vi "Curtin1_ReadWriteView.vi"(8 "X_High":dbl, 9 "X_Low":dbl, 11 "Task":enum16{"Read", "Save"}(ring)) -> (0 "X_High out":dbl, 1 "X_Low out":dbl, 3 "View":T1={"Alerts"=FALSE, "Log X Axis"=TRUE, "dB scale"=TRUE, "Averaging"=TRUE, "Fade"=0.8181818181818182, "Centroids?"=TRUE})   [LabVIEW 2022 SP3]
uses:
  Mic/Mic_Global.vi
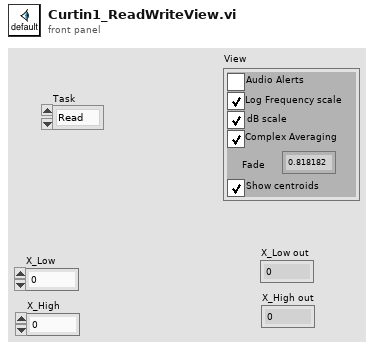
[diagram p1: front panel]
types:
  T1 = cluster{"Alerts":bool, "Log X Axis":bool, "dB scale":bool, "Averaging":bool, "Fade":dbl, "Centroids?":bool}
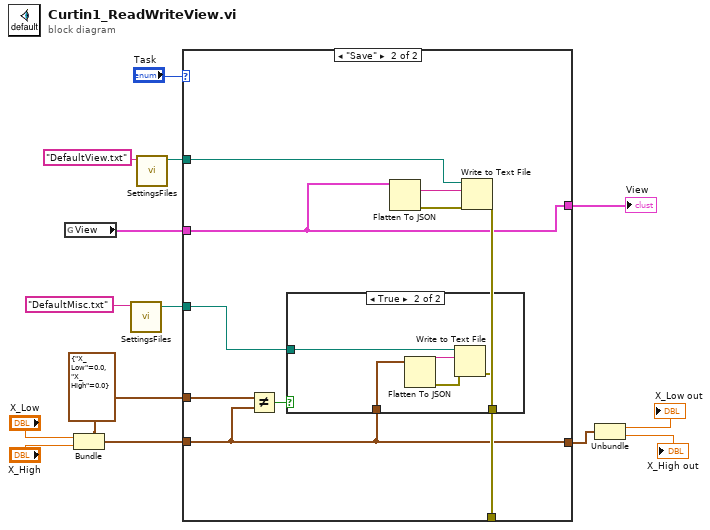
[diagram p0: block diagram]
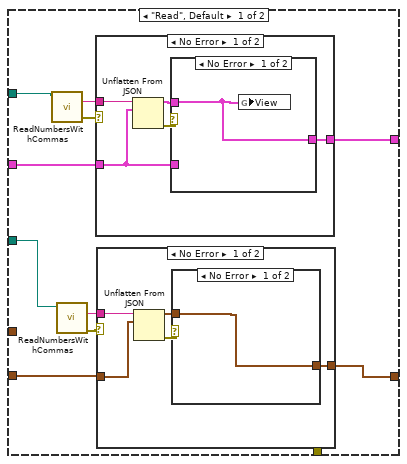
[diagram p2: hidden frame]
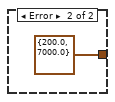
[diagram p3: hidden frame]
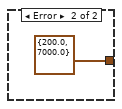
[diagram p4: hidden frame]
diagram:
  w6 = cluster{"X_Low":dbl, "X_High":dbl} {"X_Low"=0.0, "X_High"=0.0} ("output cluster")
  n1 = global read "Mic_Global.vi" "View"() -> (w10:T1)
  n2 = Bundle(cluster=w6, "X_Low"="X_Low", "X_High"="X_High") -> (w11:cluster{"X_Low":dbl, "X_High":dbl})
  n3 = call "SettingsFiles.vi"("settings file name"="DefaultMisc.txt" ("name or relative path")) -> ("file path"=w1:path)  [unwired: 9 in, 1 out]
  n4 = call "SettingsFiles.vi"("settings file name"="DefaultView.txt" ("name or relative path")) -> ("file path"=w3:path)  [unwired: 9 in, 1 out]
  n5 = case shown="\"Save\"" "Task" {
    tunnel: w3 -> [w17 w47]
    tunnel: [_ w46] -> _
    tunnel: w11 -> [w23 w42]
    tunnel: w10 -> [w24 w41]
    tunnel: w1 -> [w18 w45]
    tunnel: [w22 w42] -> w9
    tunnel: w6 -> [_ w43]
    tunnel: [w21 w41] -> w5
    frame "Read", Default {
      n6 = call "ReadNumbersWithCommas.vi"("file (use dialog)"=w17) -> ("error out"=w15:errorcluster, "text"=w16:string)  [unwired: 7 in, 2 out]
      n7 = call "ReadNumbersWithCommas.vi"("file (use dialog)"=w18) -> ("error out"=w20:errorcluster, "text"=w19:string)  [unwired: 7 in, 2 out]
      n8 = case shown="No Error" w15 {
        tunnel: w16 -> [w37 _]
        tunnel: w24 -> [w33 w40]
        tunnel: [w34 w40] -> w21
        frame No Error {
          n9 = Unflatten From JSON(JSON string=w37, type and defaults=w33) -> (value=w35:T1, error out=w36:errorcluster)  [unwired: 5 in]
          n10 = case shown="No Error" w36 {
            tunnel: w35 -> [w38 _]
            tunnel: [w38 w39] -> w34
            tunnel: w33 -> [_ w39]
            frame No Error {
              n11 = global write "Mic_Global.vi" "View"(w38) -> ()
            }
            frame Error {
            }
          }
        }
        frame Error {
        }
      }
      n12 = case shown="No Error" w20 {
        tunnel: w19 -> [w29 _]
        tunnel: w23 -> [w26 _]
        tunnel: [w25 cluster{"X_Low":dbl, "X_High":dbl} {"X_Low"=200.0, "X_High"=7000.0} ("output cluster")] -> w22
        frame No Error {
          n13 = Unflatten From JSON(JSON string=w29, type and defaults=w26) -> (value=w27:cluster{"X_Low":dbl, "X_High":dbl}, error out=w28:errorcluster)  [unwired: 5 in]
          n14 = case shown="No Error" w28 {
            tunnel: w27 -> [w30 _]
            tunnel: [w30 cluster{"X_Low":dbl, "X_High":dbl} {"X_Low"=200.0, "X_High"=7000.0} ("output cluster")] -> w25
            frame No Error {
            }
            frame Error {
            }
          }
        }
        frame Error {
        }
      }
    }
    frame "Save" {
      n15 = Not Equal?(x=w43, y=w42) -> (x != y?=w44:bool)
      n16 = case shown="True" w44 {
        tunnel: w45 -> [_ w52]
        tunnel: w42 -> [_ w51]
        tunnel: [_ w50] -> _
        frame False {
        }
        frame True {
          n17 = Flatten To JSON(anything=w51) -> (JSON string=w53:string, 11:w54:errorcluster)  [unwired: 2 in]
          n18 = Write to Text File(file (use dialog)=w52, text=w53, error in=w54) -> (error out=w50:errorcluster)  [unwired: 1 in, 2 out]
        }
      }
      n19 = Flatten To JSON(anything=w41) -> (JSON string=w49:string, 11:w48:errorcluster)  [unwired: 2 in]
      n20 = Write to Text File(file (use dialog)=w47, text=w49, error in=w48) -> (error out=w46:errorcluster)  [unwired: 1 in, 2 out]
    }
  }
  "View" <- w5
  n21 = Unbundle(w9) -> ("X_Low"=→"X_Low out":dbl, "X_High"=→"X_High out":dbl)
